vi "GT Get Follow Status.vi"(7 "pSwitchStatus":i16, 8 "error in (no error)":errorcluster caption="错误输入（无错误）", 9 "pFifoNum":i16, 10 "profile":i16, 11 "cardNum":i16) -> (0 "error out":errorcluster caption="错误输出", 1 "pFifoNum out":i16, 3 "function return":i16, 5 "pSwitchStatus out":i16)   [LabVIEW 2020, in "gts.lvlib"]
doc: "GT_API GT_GetFollowStatus(short cardNum,short profile,short *pFifoNum,short *pSwitchStatus);"
uses:
  gts.lvlib
  dll/32bit/multi_card/gts.dll
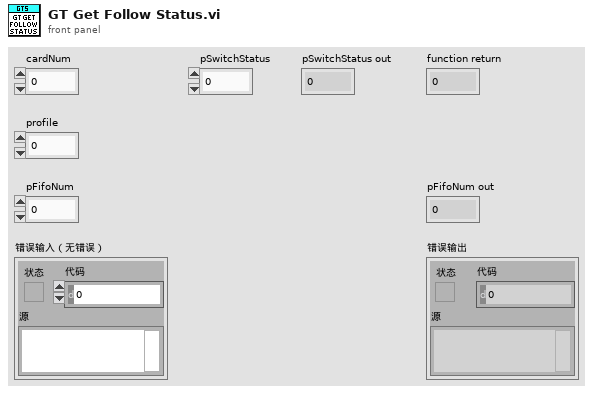
[diagram p1: front panel]
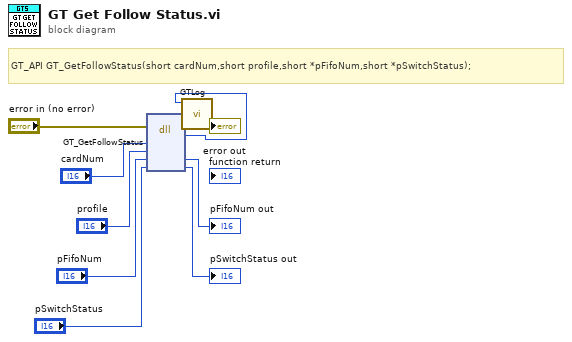
[diagram p0: block diagram]
diagram:
  # "GT_API GT_GetFollowStatus(short cardNum,short profile,short *pFifoNum,short *pSwitchStatus);"
  n1 = dll-call lib="C:/1228/dll/32bit/multi_card/gts.dll" fn="GT_GetFollowStatus"(error in="error in (no error)", "cardNum"="cardNum", "profile"="profile", "pFifoNum"="pFifoNum", "pSwitchStatus"="pSwitchStatus") -> (error out=w3:errorcluster, w1:i16, "pFifoNum"=→"pFifoNum out":i16, "pSwitchStatus"=→"pSwitchStatus out":i16)  [unwired: 4 in, 1 out]
  n2 = call "GTLog.vi"("error in (no error)"=w3, "Numeric"=w1) -> ("error out"=→"error out":errorcluster)  [unwired: 9 in]
